vi "Build message with Arguments.vi"() -> ()   [LabVIEW 2014]
uses:
  user.lib/_NEVSTOP/JKI State Machine++/_Polymophic/Build Message with Arguments(Auto Check).vi
  user.lib/_NEVSTOP/JKI State Machine++/_Polymophic/Build No-Reply Asynchronous Message with Arguments.vi
  user.lib/_NEVSTOP/JKI State Machine++/_Polymophic/Build Asynchronous Message with Arguments.vi
  user.lib/_NEVSTOP/JKI State Machine++/_Polymophic/Build Synchronous Message with Arguments.vi
  user.lib/_NEVSTOP/JKI State Machine++/_Support/Message/Parse State with Arguments String.vi
  user.lib/_NEVSTOP/JKI State Machine++/JKI State Machine++.lvlib
panel:
  in  "Tab Control":T1(tab)
  out "State with Arguments":string
  out "State with Arguments 2":string
  out "State with Arguments 3":string
  out "State with Arguments 4":string
  out "State with Arguments 5":string
  out "State with Arguments 6":string
  out "State with Arguments 7":string
  out "State with Arguments 8":string
  out "State with Arguments 9":string
  out "State with Arguments 10":string
  out "State with Arguments 11":string
  out "State with Arguments 12":string
  out "State with Arguments 13":string
  out "State with Arguments 14":string
  out "State with Arguments 15":string
  out "State with Arguments 16":string
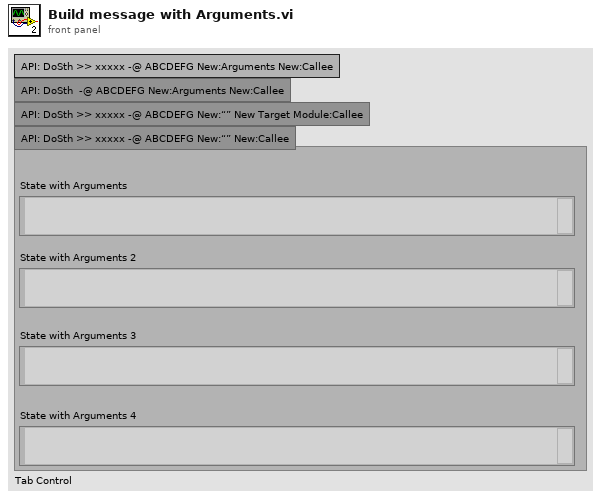
[diagram p1: front panel]
types:
  T1 = enum32{"API: DoSth >> xxxxx -@ ABCDEFG New:Arguments New:Callee", "API: DoSth  -@ ABCDEFG New:Arguments New:Callee", "API: DoSth >> xxxxx -@ ABCDEFG New:“” New Target Module:Callee", "API: DoSth >> xxxxx -@ ABCDEFG New:“” New:Callee"}
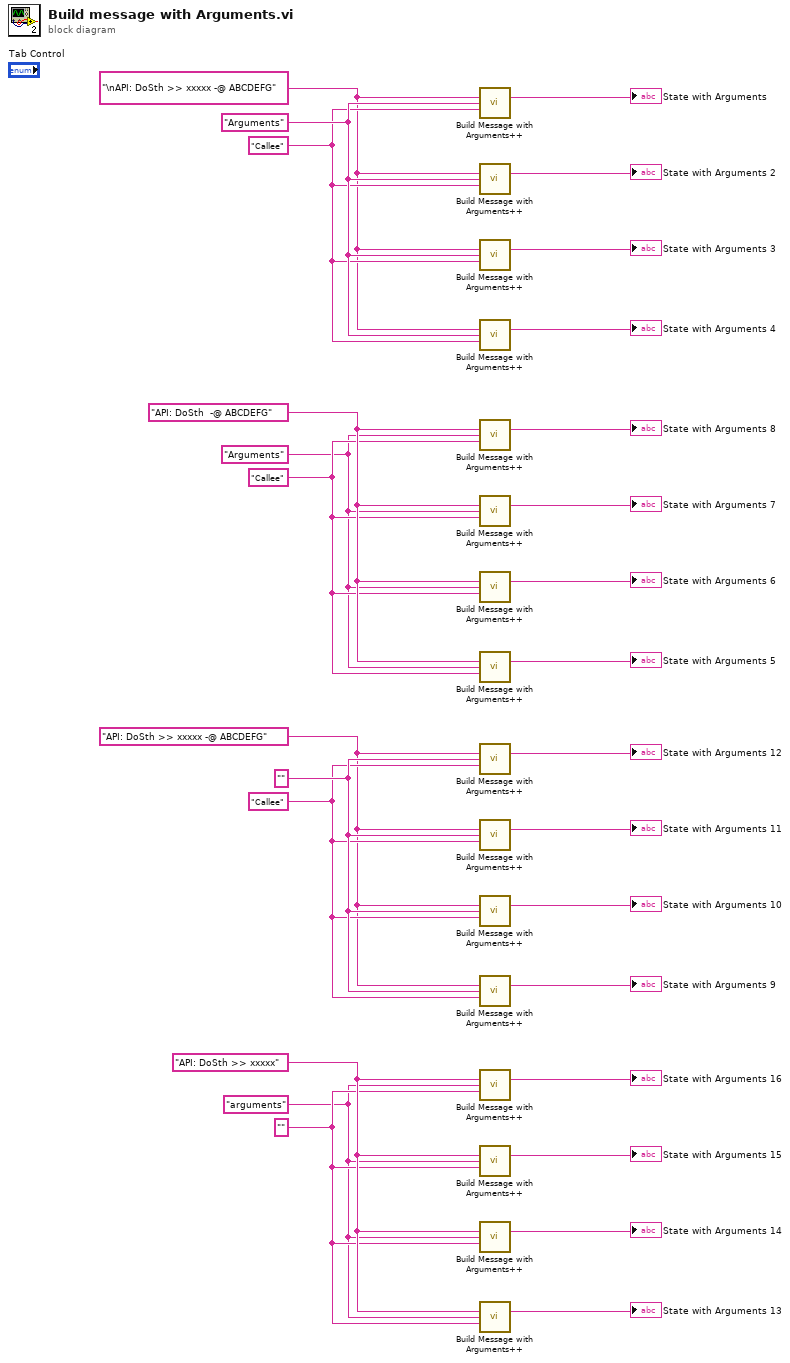
[diagram p0: block diagram]
diagram:
  w6 = "" ("State with Arguments")
  w5 = "arguments" ("State with Arguments")
  w7 = "API: DoSth >> xxxxx" ("State with Arguments")
  w9 = "Callee" ("State with Arguments")
  w10 = "" ("State with Arguments")
  w8 = "API: DoSth >> xxxxx -@ ABCDEFG" ("State with Arguments")
  w20 = "Callee" ("State with Arguments")
  w19 = "Arguments" ("State with Arguments")
  w21 = "API: DoSth  -@ ABCDEFG" ("State with Arguments")
  w23 = "Callee" ("State with Arguments")
  w24 = "Arguments" ("State with Arguments")
  w22 = "\nAPI: DoSth >> xxxxx -@ ABCDEFG" ("State with Arguments")
  n1 = call-poly "Build Message with Arguments++.vi"("State with Arguments"=w22, "Arguments (\"\")"=w24, "Target Module (\"\")"=w23) -> ("State with Arguments"=→"State with Arguments":string)  [unwired: 12 in]
  n2 = call-poly "Build Message with Arguments++.vi"("State with Arguments"=w22, "Arguments (\"\")"=w24, "Target Module (\"\")"=w23) -> ("State with Arguments"=→"State with Arguments 2":string)  [unwired: 12 in]
  n3 = call-poly "Build Message with Arguments++.vi"("State with Arguments"=w22, "Arguments (\"\")"=w24, "Target Module (\"\")"=w23) -> ("State with Arguments"=→"State with Arguments 3":string)  [unwired: 12 in]
  n4 = call-poly "Build Message with Arguments++.vi"("State with Arguments"=w22, "Arguments (\"\")"=w24, "Target Module (\"\")"=w23) -> ("State with Arguments"=→"State with Arguments 4":string)  [unwired: 12 in]
  n5 = call-poly "Build Message with Arguments++.vi"("State with Arguments"=w21, "Arguments (\"\")"=w19, "Target Module (\"\")"=w20) -> ("State with Arguments"=→"State with Arguments 8":string)  [unwired: 12 in]
  n6 = call-poly "Build Message with Arguments++.vi"("State with Arguments"=w21, "Arguments (\"\")"=w19, "Target Module (\"\")"=w20) -> ("State with Arguments"=→"State with Arguments 7":string)  [unwired: 12 in]
  n7 = call-poly "Build Message with Arguments++.vi"("State with Arguments"=w21, "Arguments (\"\")"=w19, "Target Module (\"\")"=w20) -> ("State with Arguments"=→"State with Arguments 6":string)  [unwired: 12 in]
  n8 = call-poly "Build Message with Arguments++.vi"("State with Arguments"=w21, "Arguments (\"\")"=w19, "Target Module (\"\")"=w20) -> ("State with Arguments"=→"State with Arguments 5":string)  [unwired: 12 in]
  n9 = call-poly "Build Message with Arguments++.vi"("State with Arguments"=w8, "Arguments (\"\")"=w10, "Target Module (\"\")"=w9) -> ("State with Arguments"=→"State with Arguments 12":string)  [unwired: 12 in]
  n10 = call-poly "Build Message with Arguments++.vi"("State with Arguments"=w8, "Arguments (\"\")"=w10, "Target Module (\"\")"=w9) -> ("State with Arguments"=→"State with Arguments 11":string)  [unwired: 12 in]
  n11 = call-poly "Build Message with Arguments++.vi"("State with Arguments"=w8, "Arguments (\"\")"=w10, "Target Module (\"\")"=w9) -> ("State with Arguments"=→"State with Arguments 10":string)  [unwired: 12 in]
  n12 = call-poly "Build Message with Arguments++.vi"("State with Arguments"=w8, "Arguments (\"\")"=w10, "Target Module (\"\")"=w9) -> ("State with Arguments"=→"State with Arguments 9":string)  [unwired: 12 in]
  n13 = call-poly "Build Message with Arguments++.vi"("State with Arguments"=w7, "Arguments (\"\")"=w5, "Target Module (\"\")"=w6) -> ("State with Arguments"=→"State with Arguments 16":string)  [unwired: 12 in]
  n14 = call-poly "Build Message with Arguments++.vi"("State with Arguments"=w7, "Arguments (\"\")"=w5, "Target Module (\"\")"=w6) -> ("State with Arguments"=→"State with Arguments 15":string)  [unwired: 12 in]
  n15 = call-poly "Build Message with Arguments++.vi"("State with Arguments"=w7, "Arguments (\"\")"=w5, "Target Module (\"\")"=w6) -> ("State with Arguments"=→"State with Arguments 14":string)  [unwired: 12 in]
  n16 = call-poly "Build Message with Arguments++.vi"("State with Arguments"=w7, "Arguments (\"\")"=w5, "Target Module (\"\")"=w6) -> ("State with Arguments"=→"State with Arguments 13":string)  [unwired: 12 in]
